vi "Make Holonomic.vi"(6 "Drive Type":T2, 7 "Trajectory Data In":T1(array[cluster]), 9 "WayPoints":cluster{"x":dbl, "y":dbl, "th":dbl}[](array[cluster]), 10 "Sample Period (s)":dbl, 11 "Angular Limits":T3={"Velocity (deg/s)"=6.0, "Accel (deg/s^2)"=15.0, "Jerk (deg/s^3)"=150.0} {"Jerk (deg/s^3)" min=0.0 step=1.0; "Accel (deg/s^2)" min=0.0; "Velocity (deg/s)" min=0.0}) -> (2 "Headings":dbl[](array[numeric]), 3 "Trajectory Data Out":T1(array[cluster]))   [LabVIEW 2025]
uses:
  Types/Angluar Limits.ctl
  Types/Drive Type.ctl
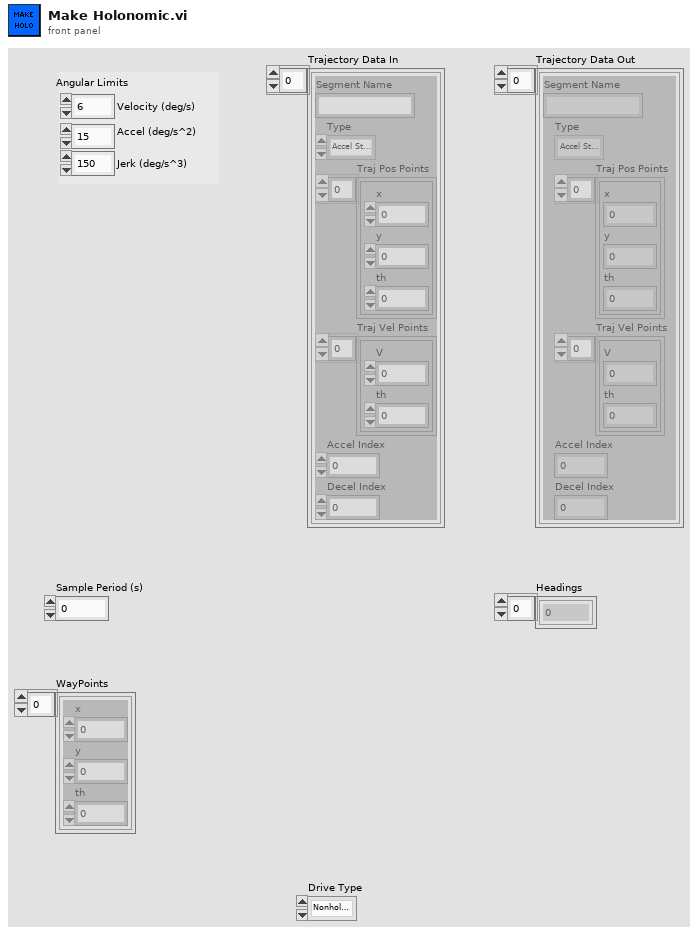
[diagram p1: front panel]
types:
  T1 = cluster{"Segment Name":string, "Type":enum16{"Accel Straight", "Const Straight", "Blend", "Circle"}, "Traj Pos Points":cluster{"x":dbl, "y":dbl, "th":dbl}[], "Traj Vel Points":cluster{"V":dbl, "th":dbl}[], "Accel Index":i32, "Decel Index":i32}[]
  T2 = typedef "Drive Type.ctl" = enum16{"Nonholonomic", "Holonomic"}
  T3 = typedef "Angluar Limits.ctl" = cluster{"Velocity (deg/s)":dbl, "Accel (deg/s^2)":dbl, "Jerk (deg/s^3)":dbl}
  T4 = cluster{"Segment Name":string, "Type":enum16{"Accel Straight", "Const Straight", "Blend", "Circle"}, "Traj Pos Points":cluster{"x":dbl, "y":dbl, "th":dbl}[], "Traj Vel Points":cluster{"V":dbl, "th":dbl}[], "Accel Index":i32, "Decel Index":i32}
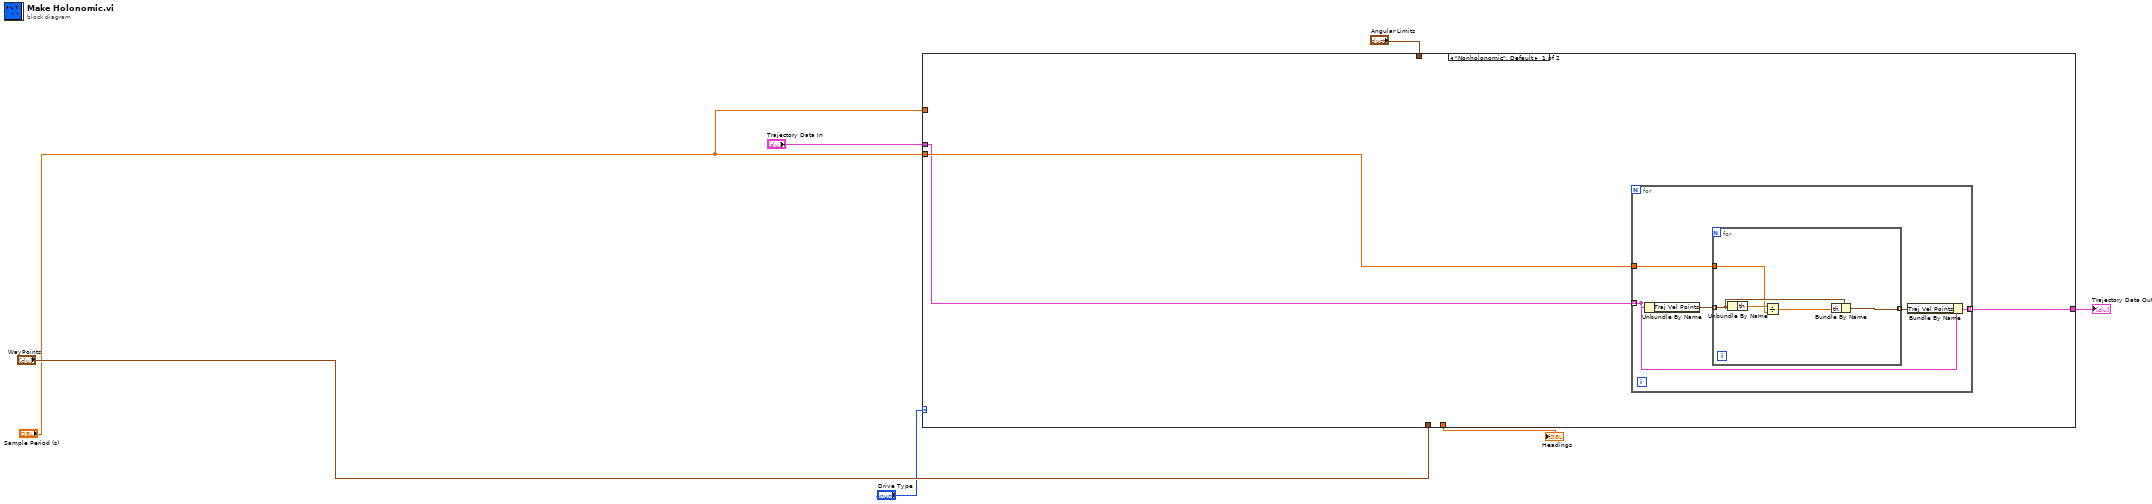
[diagram p0: block diagram]
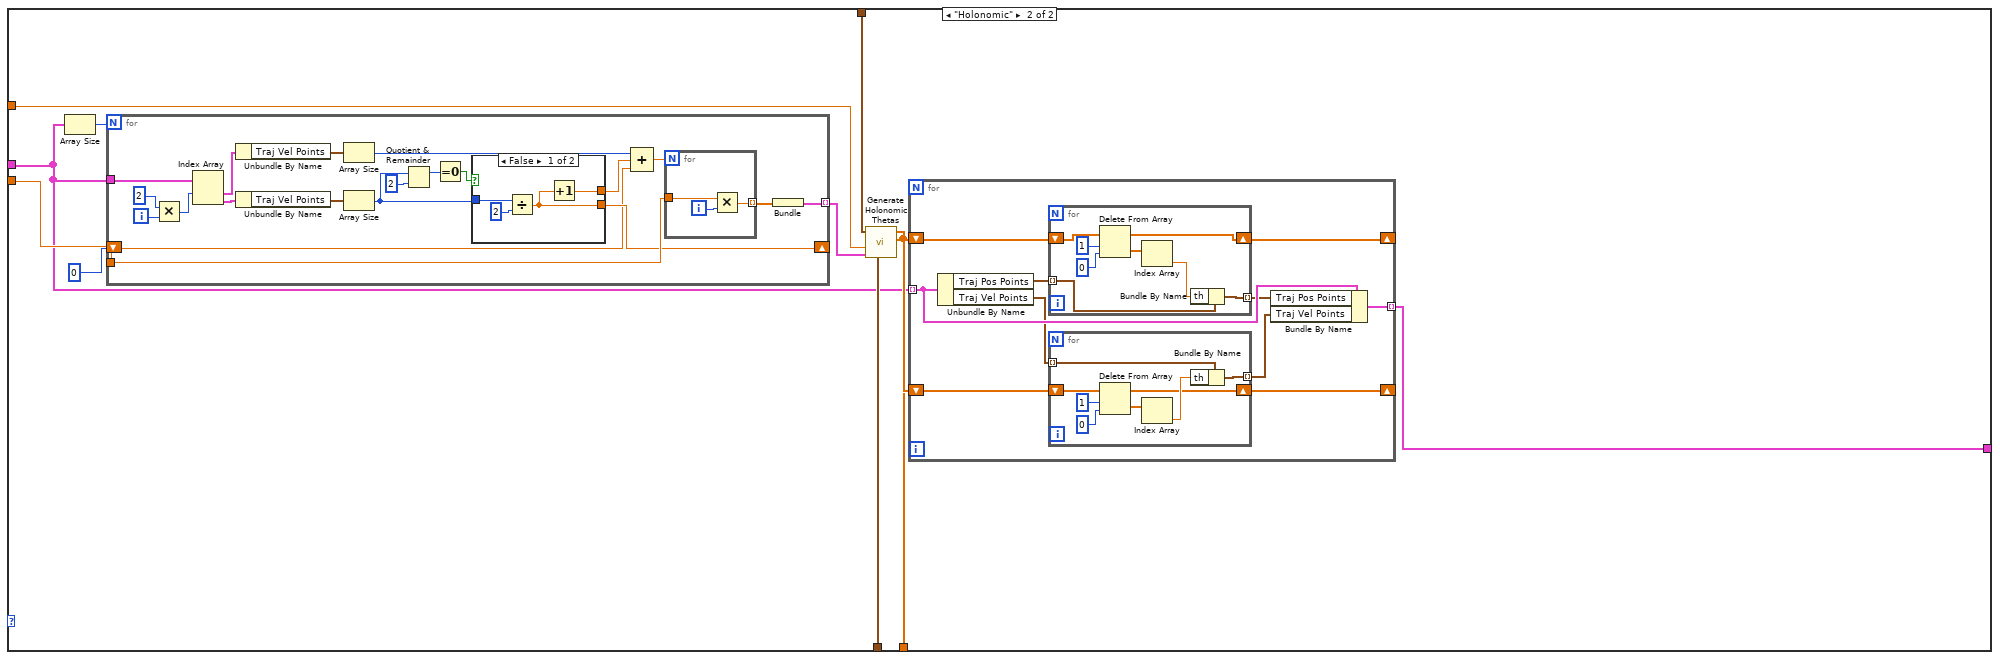
[diagram p2: hidden frame]
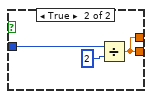
[diagram p3: hidden frame]
diagram:
  n1 = case shown="\"Nonholonomic\", Default" "Drive Type" {
    tunnel: [w8 w31] -> w7
    tunnel: "Sample Period (s)" -> [_ w29]
    tunnel: "Angular Limits" -> [_ w28]
    tunnel: "Sample Period (s)" -> [w10 w30]
    tunnel: [_ w26] -> w1
    tunnel: "Trajectory Data In" -> [w9 w21]
    tunnel: "WayPoints" -> [_ w25]
    frame "Nonholonomic", Default {
      n2 = for {
        tunnel: [w13] -> w8 mode=indexing
        tunnel: w10 -> [w12]
        tunnel: w9 -> [w11] mode=indexing
        n3 = Unbundle By Name(w11) -> ("Traj Vel Points"=w15:cluster{"V":dbl, "th":dbl}[])
        n4 = for {
          tunnel: w15 -> [w19] mode=indexing
          tunnel: [w17] -> w14 mode=indexing
          tunnel: w12 -> [w16]
          n5 = Unbundle By Name(w19) -> ("th"=w20:dbl)
          n6 = Divide(x=w20, y=w16) -> (x/y=w18:dbl)
          n7 = Bundle By Name(cluster=w19, "th"=w18) -> (w17:cluster{"V":dbl, "th":dbl})
        }
        n8 = Bundle By Name(cluster=w11, "Traj Vel Points"=w14) -> (w13:T4)
      }
    }
    frame "Holonomic" {
      n9 = Array Size(array=w21) -> (size(s)=w22:i32)
      n10 = for {
        N: w22 -> [_]
        tunnel: w21 -> [w50]
        tunnel: w30 -> [w51]
        shift-right: [w44] -> _
        shift-left: 0 -> [w41]
        tunnel: [w42] -> w23 mode=indexing
        i -> [w34]
        n11 = Multiply(x=2, y=w34) -> (x*y=w32:i32)
        n12 = Index Array(array=w50, index #1=w32) -> (element #1=w49:T4, element #2=w47:T4)  [unwired: 1 in]
        n13 = Unbundle By Name(w49) -> ("Traj Vel Points"=w48:cluster{"V":dbl, "th":dbl}[])
        n14 = Unbundle By Name(w47) -> ("Traj Vel Points"=w46:cluster{"V":dbl, "th":dbl}[])
        n15 = Array Size(array=w48) -> (size(s)=w45:i32)
        n16 = Array Size(array=w46) -> (size(s)=w39:i32)
        n17 = Quotient & Remainder(x=w39, y=2) -> (x-y*floor(x/y)=w40:i32)  [unwired: 1 out]
        n18 = Equal To 0?(x=w40) -> (x = 0?=w37:bool)
        n19 = case shown="False" w37 {
          tunnel: w39 -> [w52 w58]
          tunnel: [w53 w56] -> w44
          tunnel: [w54 w56] -> w36
          frame False {
            n20 = Divide(x=w52, y=2) -> (x/y=w53:dbl)
            n21 = Increment(x=w53) -> (x+1=w54:dbl)
          }
          frame True {
            n22 = Divide(x=w58, y=2) -> (x/y=w56:dbl)
          }
        }
        n23 = Compound Arithmetic op=ADD(w45, w36, w41) -> (w35:dbl)
        n24 = for {
          N: w35 -> [_]
          tunnel: w51 -> [w60]
          tunnel: [w59] -> w43 mode=indexing
          i -> [w61]
          n25 = Multiply(x=w60, y=w61) -> (x*y=w59:dbl)
        }
        n26 = Bundle(w43) -> (w42:cluster{dbl[]})  [unwired: 1 in]
      }
      n27 = call "Generate Holonomic Thetas.vi"("WayPoints"=w25, "time unflat"=w23, "dt"=w29, "Angular Limits"=w28) -> ("X"=w26:dbl[], "V"=w27:dbl[])  [unwired: 6 in]
      n28 = for {
        tunnel: w21 -> [w70] mode=indexing
        shift-right: [w62] -> _
        shift-left: w26 -> [w63]
        shift-right: [w64] -> _
        shift-left: w27 -> [w65]
        tunnel: [w66] -> w31 mode=indexing
        n29 = Unbundle By Name(w70) -> ("Traj Pos Points"=w71:cluster{"x":dbl, "y":dbl, "th":dbl}[], "Traj Vel Points"=w68:cluster{"V":dbl, "th":dbl}[])
        n30 = for {
          tunnel: w71 -> [w87] mode=indexing
          tunnel: [w86] -> w69 mode=indexing
          shift-right: [w81] -> w62
          shift-left: w63 -> [w84]
          n31 = Delete From Array(array=w84, length=1, index=0) -> (deleted portion=w85:dbl[], array with subset deleted=w81:dbl[])
          n32 = Index Array(array=w85) -> (element=w82:dbl)  [unwired: 1 in]
          n33 = Bundle By Name(cluster=w87, "th"=w82) -> (w86:cluster{"x":dbl, "y":dbl, "th":dbl})
        }
        n34 = for {
          tunnel: w68 -> [w79] mode=indexing
          tunnel: [w78] -> w67 mode=indexing
          shift-right: [w74] -> w64
          shift-left: w65 -> [w77]
          n35 = Delete From Array(array=w77, length=1, index=0) -> (deleted portion=w73:dbl[], array with subset deleted=w74:dbl[])
          n36 = Index Array(array=w73) -> (element=w75:dbl)  [unwired: 1 in]
          n37 = Bundle By Name(cluster=w79, "th"=w75) -> (w78:cluster{"V":dbl, "th":dbl})
        }
        n38 = Bundle By Name(cluster=w70, "Traj Pos Points"=w69, "Traj Vel Points"=w67) -> (w66:T4)
      }
    }
  }
  "Trajectory Data Out" <- w7
  "Headings" <- w1
